vi "traffic control sms IO.vi"(1 "state":u16(ring) items=["Init", "Write", "Read", "Close"], 2 "eventch":string, 9 "enable sms":bool, 11 "error in":errorcluster, 13 "sms":bool[](array[boolean])) -> (6 "sms indikator":bool[](array[boolean]), 15 "error out":errorcluster)   [LabVIEW 2017]
uses:
  <vilib>/DAQmx/write.llb/DAQmx Write (Digital 1D Bool NChan 1Samp 1Line).vi
  <vilib>/DAQmx/read.llb/DAQmx Read (Digital Bool 1Line 1Point).vi
  <vilib>/DAQmx/create/channels.llb/DAQmx Create Channel (DO-Digital Output).vi
  <vilib>/DAQmx/miscellaneous.llb/DAQmx Fill In Error Info.vi
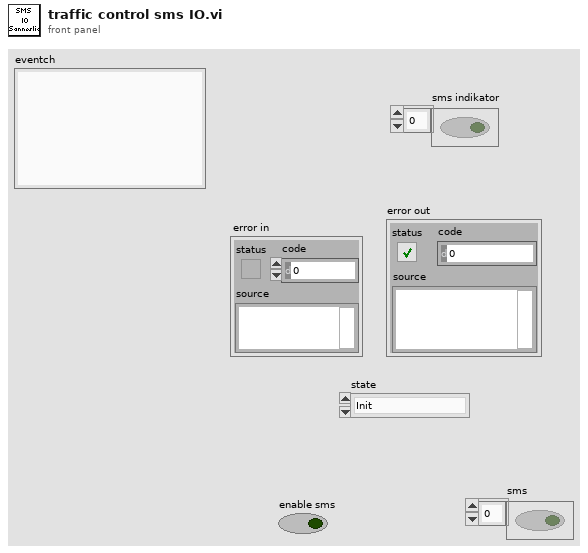
[diagram p1: front panel]
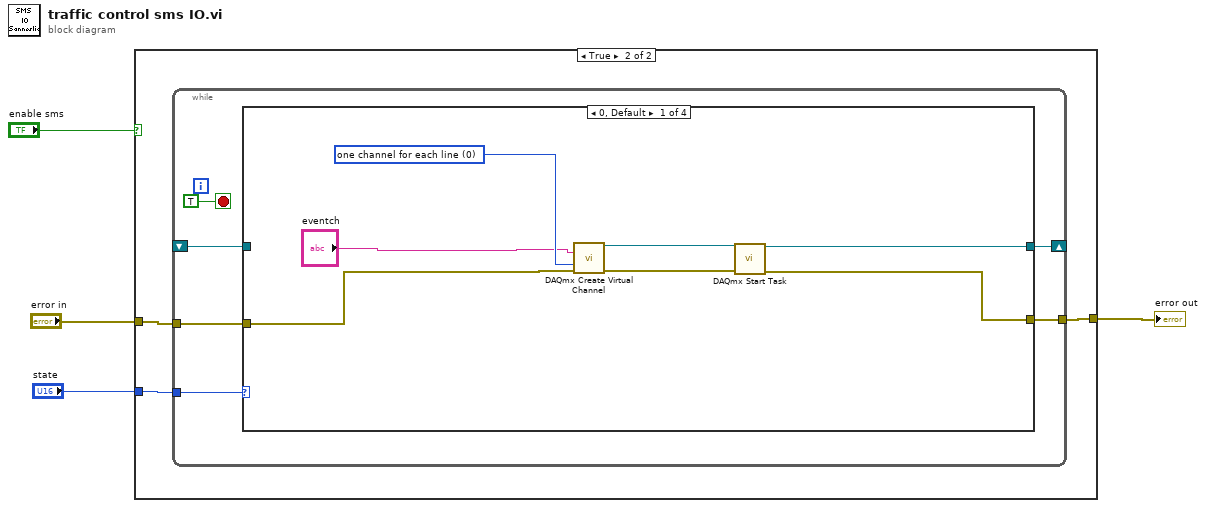
[diagram p0: block diagram]
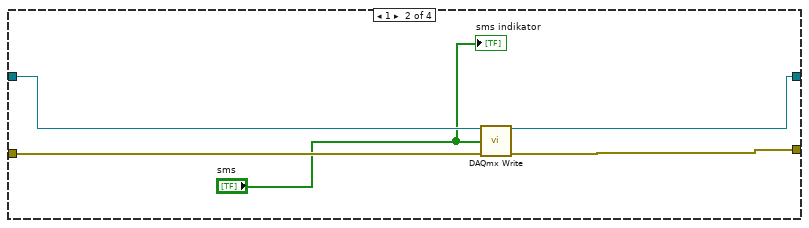
[diagram p3: hidden frame]
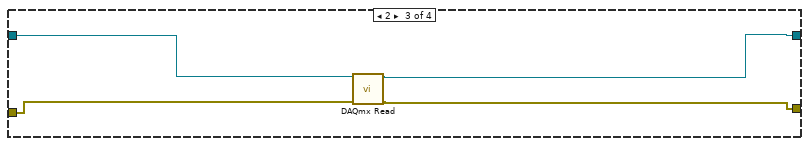
[diagram p4: hidden frame]
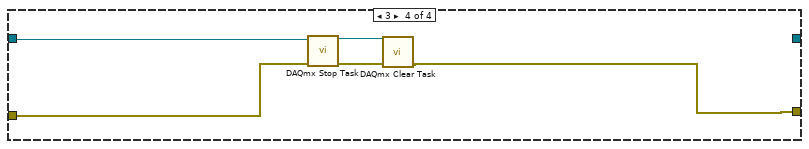
[diagram p5: hidden frame]
diagram:
  n1 = case shown="True" "enable sms" {
    tunnel: "state" -> [_ w8]
    tunnel: "error in" -> [w5 w6]
    tunnel: [w5 w7] -> w2
    frame False {
    }
    frame True {
      n2 = while {
        tunnel: w8 -> [w13]
        tunnel: [w14] -> w7
        shift-right: [w12] -> _
        shift-left: _ -> [w11]
        tunnel: w6 -> [w10]
        stop <- TRUE stop-if-true
        n3 = case shown="0, Default" w13 {
          tunnel: [w19 w25 w27 w32] -> w14
          tunnel: [w18 w26 w30 _] -> w12
          tunnel: w11 -> [_ w24 w29 w33]
          tunnel: w10 -> [w15 w23 w28 w31]
          frame 0, Default {
            w17 = 0 items=["one channel for each line", "one channel for all lines"] ("line grouping")
            n4 = call-poly <vilib>:"DAQmx Create Virtual Channel.vi"("lines"="eventch", "line grouping"=w17, "error in"=w15) -> ("task out"=w21:refnum<k21>, "error out"=w20:errorcluster)  [unwired: 11 in]
            n5 = call <vilib>:"DAQmx Start Task.vi"("task/channels in"=w21, "error in"=w20) -> ("task out"=w18:refnum<k21>, "error out"=w19:errorcluster)  [unwired: 12 in]
          }
          frame 1 {
            n6 = call-poly <vilib>:"DAQmx Write.vi"("task/channels in"=w24, "data"="sms", "error in"=w23) -> ("task out"=w26:refnum<k21>, "error out"=w25:errorcluster)  [unwired: 10 in, 1 out]
            "sms indikator" <- "sms"
          }
          frame 2 {
            n7 = call-poly <vilib>:"DAQmx Read.vi"("task/channels in"=w29, "error in"=w28) -> ("task out"=w30:refnum<k21>, "error out"=w27:errorcluster)  [unwired: 11 in, 1 out]
          }
          frame 3 {
            n8 = call <vilib>:"DAQmx Stop Task.vi"("task/channels in"=w33, "error in"=w31) -> ("task out"=w34:refnum<k21>, "error out"=w35:errorcluster)  [unwired: 12 in]
            n9 = call <vilib>:"DAQmx Clear Task.vi"("task in"=w34, "error in"=w35) -> ("error out"=w32:errorcluster)  [unwired: 13 in]
          }
        }
      }
    }
  }
  "error out" <- w2
